vi "AxisWriteValues_Write.vi"(1 "AxisWriteValuesIN":T1={"AxisTarget"=0.0, "AxisTargetVel"=1.0, "AxisStartReq"=FALSE, "AxisStopReq"=FALSE, "AxisClearReq"=FALSE, "AxisMovetype"=FALSE, "AxisMotorON"=FALSE, "MoveModeControl"=0, "AxisHomingVel"=1.0, "AxisAccDecc"=30.0} {"MoveModeControl" items=["Absolute"=1, "Relative"=2, "Velocity"=3, "Homing"=4, "none"=0]}, 2 "AxisNo":u16) -> ()   [LabVIEW 2020, in "SMCD14_lib.lvlib"]
uses:
  SMCD14_lib.lvlib
  AxisWriteValues_typedef.ctl
  Globals.vi
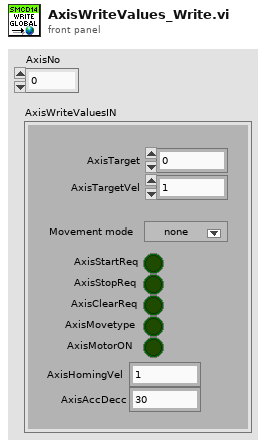
[diagram p1: front panel]
types:
  T1 = typedef "SMCD14_lib.lvlib/AxisWriteValues_typedef.ctl" = cluster{"AxisTarget":dbl, "AxisTargetVel":dbl, "AxisStartReq":bool, "AxisStopReq":bool, "AxisClearReq":bool, "AxisMovetype":bool, "AxisMotorON":bool, "MoveModeControl":u16, "AxisHomingVel":dbl, "AxisAccDecc":dbl}
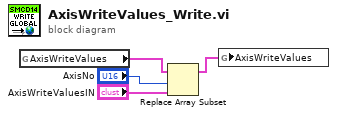
[diagram p0: block diagram]
diagram:
  n1 = global read "Globals.vi" "AxisWriteValues"() -> (w4:T1[])
  n2 = Replace Array Subset(array=w4, new element="AxisWriteValuesIN", index="AxisNo") -> (w3:T1[])
  n3 = global write "Globals.vi" "AxisWriteValues"(w3) -> ()
